vi "osd_get_data.vi"(4 "bypara":u8, 5 "COM":bool, 6 "byIndex":u8, 7 "VISA name":refnum<visa-resource-name>, 10 "bySubcmd":u8, 11 "byCmd":u8) -> (2 "data out":u8[](array[numeric]), 3 "return":i32)   [LabVIEW 2016]
panel:
  in  "vdcmd_info_osd_t":T1
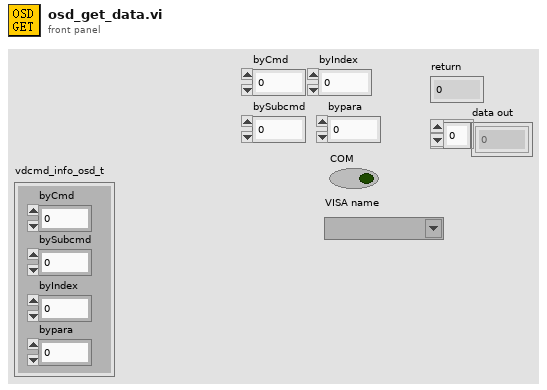
[diagram p1: front panel]
types:
  T1 = cluster{"byCmd":u8, "bySubcmd":u8, "byIndex":u8, "bypara":u8}
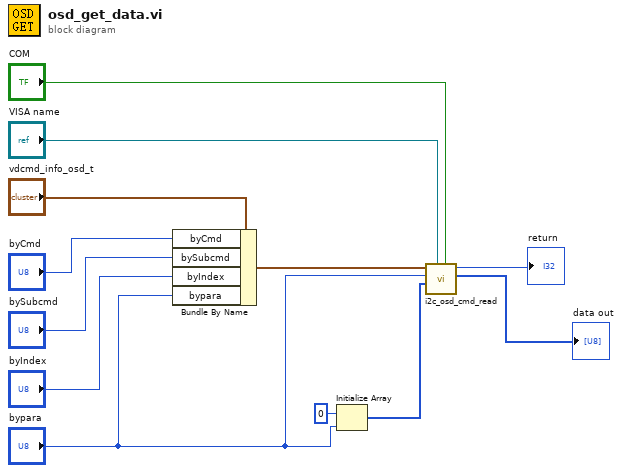
[diagram p0: block diagram]
diagram:
  n1 = Bundle By Name(cluster="vdcmd_info_osd_t", "byCmd"="byCmd", "bySubcmd"="bySubcmd", "byIndex"="byIndex", "bypara"="bypara") -> (w8:T1)
  n2 = Initialize Array(u8 0 ("element"), "bypara") -> (w1:u8[])
  n3 = call "i2c_osd_cmd_read.vi"("COM"="COM", "VISA name"="VISA name", "data in"=w1, "byDataLen"="bypara", "vdcmd_info_osd_t"=w8) -> ("data out"=→"data out":u8[], "return"=→"return":i32)  [unwired: 5 in]
